vi "EOL CAN_Get Seed_and_Key_FBL_C70.vi"(7 "Rx Arbitration Id":u32=402522244 format="%.0x", 8 "Error in":errorcluster, 10 "Read Session in":refnum<k21>, 11 "Write Session in":refnum<k21>) -> (0 "Error out":errorcluster, 2 "Response Good?":bool, 3 "TxRx Data":string[][](array[string]))   [LabVIEW 2018]
uses:
  <vilib>/xnet/xnet.llb/XNET Frame CAN.ctl
  <vilib>/xnet/xnet.llb/XNET Frame Type CAN.ctl
panel:
  out "Key":u32[](array[numeric]) format="%x"
  in  "Seed message":u8[](array[numeric])=[6, 103, 1, 36, 34, 32, 31, 0] format="%x"
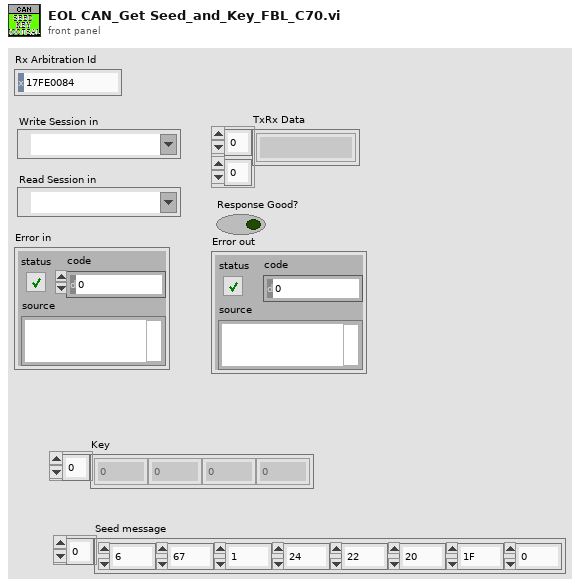
[diagram p1: front panel]
types:
  T1 = typedef "XNET Frame CAN.ctl" = cluster{"timestamp":timestamp, "payload":u8[], "identifier":u32, "type":T2, "extended?":bool, "echo?":bool}
  T2 = typedef "XNET Frame Type CAN.ctl" = u8
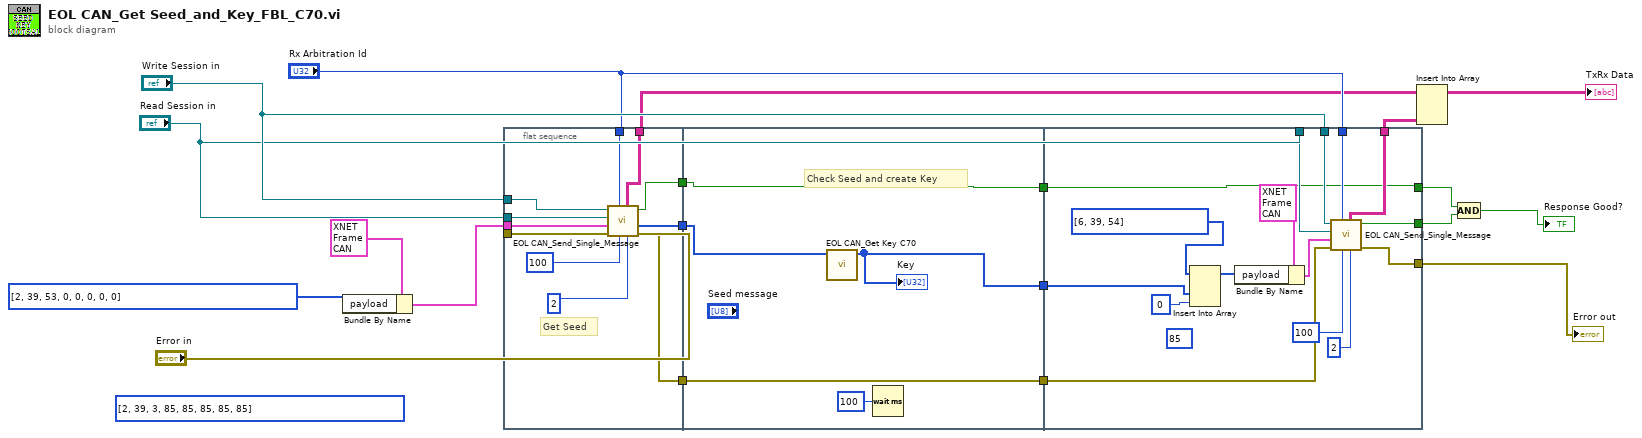
[diagram p0: block diagram]
diagram:
  (unwired) u8[] [2, 39, 3, 85, 85, 85, 85, 85] ("Transmit Data 2")
  n1 = Bundle By Name(cluster=T1 {"timestamp"=timestamp(0 s since 1904-01-01), "payload"=[2, 39, 3, 85, 85, 85, 85, 85], "identifier"=1859, "type"=8, "extended?"=FALSE, "echo?"=FALSE} ("Tx CAN frame"), "payload"=u8[] [2, 39, 53, 0, 0, 0, 0, 0] ("Transmit Data 2")) -> (w12:T1)
  n2 = flat-sequence {
    tunnel: [w30] -> w7
    tunnel: w12 -> [w29]
    tunnel: "Read Session in" -> [w28]
    tunnel: "Write Session in" -> [w27]
    tunnel: "Error in" -> [w26]
    tunnel: "Rx Arbitration Id" -> [w24]
    tunnel: [w31] -> w20
    tunnel: [w25] -> w19
    tunnel: [w23] -> w18
    tunnel: w20 -> [w35]
    tunnel: w19 -> [w36]
    tunnel: [w36] -> w17
    tunnel: w18 -> [w32]
    tunnel: [w33] -> w16
    tunnel: [w35] -> w15
    tunnel: w17 -> [w52]
    tunnel: w16 -> [w44]
    tunnel: "Write Session in" -> [w49]
    tunnel: "Read Session in" -> [w48]
    tunnel: "Rx Arbitration Id" -> [w47]
    tunnel: [w46] -> w6
    tunnel: [w41] -> w2
    tunnel: w15 -> [w40]
    tunnel: [w40] -> w3
    tunnel: [w39] -> w1
    frame #0 {
      # "Get Seed"
      n3 = call "EOL CAN_Send_Single_Message.vi"("Retries"=2, "Msg Wait Time"=u32 100, "Rx Arbitration Id"=w24, "Error in"=w26, "Tx CAN frame"=w29, "Read Session in"=w28, "Write Session in"=w27) -> ("Error out"=w25:errorcluster, "Rx Message"=w23:u8[], "Response Good?"=w31:bool, "TxRx Data"=w30:string[][])  [unwired: 1 out]
    }
    frame #1 {
      # "Check Seed and create Key"
      n4 = call "EOL CAN_Get Key C70.vi"("Seed message"=w32) -> ("Key"=w33:u32[])  [unwired: 10 in]
      "Key" <- w33
      n5 = Wait (ms)(milliseconds to wait=u32 100) -> ()  [unwired: 1 out]
    }
    frame #2 {
      (unwired) u8 85 ("new element/subarray")
      n6 = Insert Into Array(array=u8[] [6, 39, 54] ("payload"), new element #1=w44, new element #2=u8 0 ("new element/subarray")) -> (w42:u8[])  [unwired: 1 in]
      n7 = Bundle By Name(cluster=T1 {"timestamp"=timestamp(0 s since 1904-01-01), "payload"=[2, 39, 3, 85, 85, 85, 85, 85], "identifier"=1859, "type"=8, "extended?"=FALSE, "echo?"=FALSE} ("Tx CAN frame"), "payload"=w42) -> (w50:T1)
      n8 = call "EOL CAN_Send_Single_Message.vi"("Retries"=2, "Msg Wait Time"=u32 100, "Rx Arbitration Id"=w47, "Error in"=w52, "Tx CAN frame"=w50, "Read Session in"=w48, "Write Session in"=w49) -> ("Error out"=w39:errorcluster, "Response Good?"=w41:bool, "TxRx Data"=w46:string[][])  [unwired: 2 out]
    }
  }
  n9 = Insert Into Array(array=w7, new element=w6) -> (→"TxRx Data":string[][])  [unwired: 2 in]
  n10 = Compound Arithmetic op=AND(w3, w2) -> (→"Response Good?":bool)
  "Error out" <- w1
